vi "Excel_average.vi"(4 "Save?":bool, 6 "1_IL,0_uL":bool, 7 "KG20":dbl[](array[numeric]), 8 "error in (no error)":errorcluster, 9 "Test?":bool, 10 "Report path in":path, 11 "report in":refnum<class "NI_report.lvclass">) -> (0 "error out":errorcluster, 2 "Report path out":path, 3 "report out":refnum<class "NI_report.lvclass">)   [LabVIEW 2015]
doc: "输出电流因数的平均值和与1.125差值"
uses:
  <vilib>/Utility/NIReport.llb/NI_report.lvclass
  <vilib>/addons/_office/NI_ReportGenerationToolkit.lvlib
panel:
  in  "start(-1,-1)":cluster{"row":i32, "column":i32}
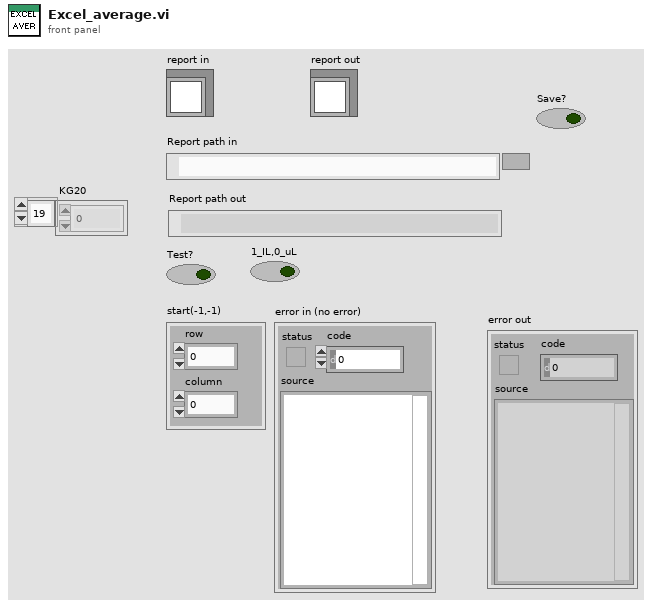
[diagram p1: front panel]
types:
  T1 = enum16{"Standard Report", "HTML", "Word", "Excel"}
  T2 = enum16{"maximized", "minimized", "normal", "no change"}
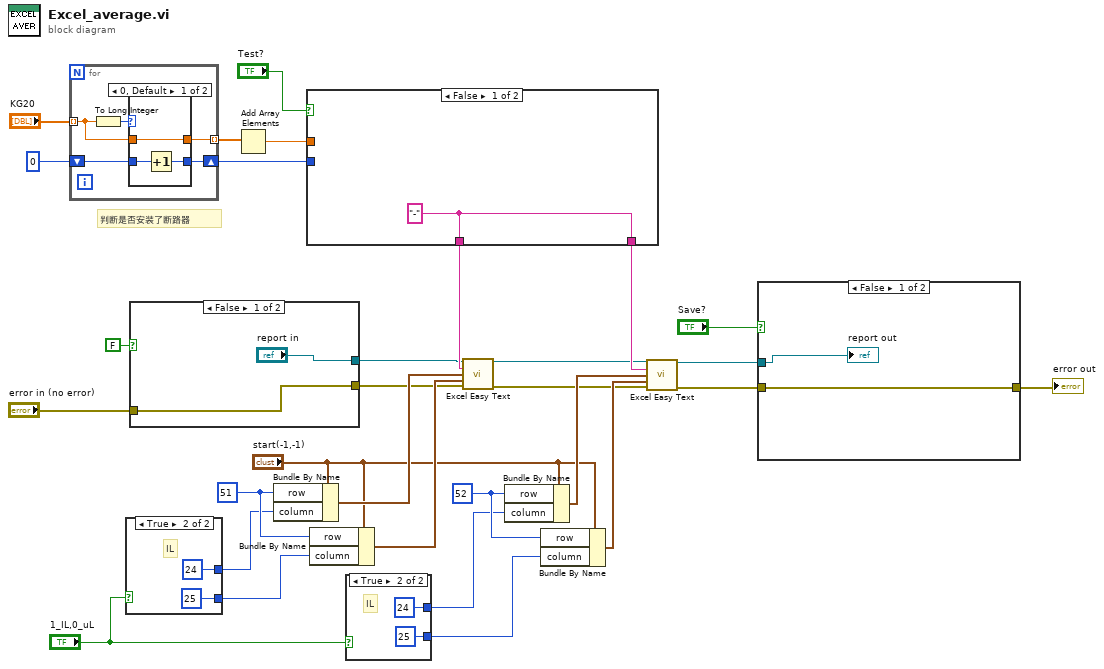
[diagram p0: block diagram]
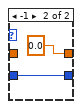
[diagram p2: hidden frame]
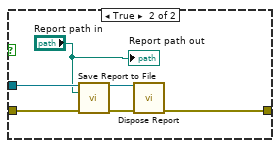
[diagram p3: hidden frame]
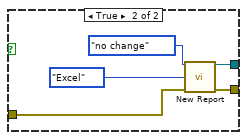
[diagram p4: hidden frame]
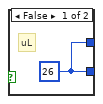
[diagram p5: hidden frame]
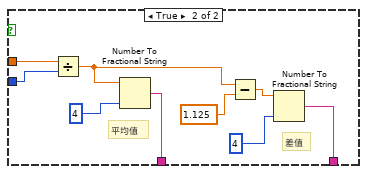
[diagram p6: hidden frame]
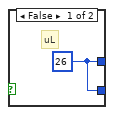
[diagram p7: hidden frame]
diagram:
  w23 = 52 ("row")
  w26 = 51 ("row")
  # "判断是否安装了断路器"
  n1 = for {
    tunnel: "KG20" -> [w33] mode=indexing
    shift-right: [w34] -> w3
    shift-left: 0 -> [w35]
    tunnel: [w32] -> w1 mode=indexing
    n2 = To Long Integer(number=w33) -> (32bit integer=w31:i32)
    n3 = case shown="0, Default" w31 {
      tunnel: w35 -> [w38 w39]
      tunnel: [w36 w39] -> w34
      tunnel: [w37 0.0] -> w32
      tunnel: w33 -> [w37 _]
      frame 0, Default {
        n4 = Increment(x=w38) -> (x+1=w36:i32)
      }
      frame -1 {
      }
    }
  }
  n5 = case shown="True" "1_IL,0_uL" {
    tunnel: [w41 24 ("column")] -> w16
    tunnel: [w41 25 ("column")] -> w15
    frame False {
      w41 = 26 ("column")
      # "uL"
    }
    frame True {
      # "IL"
    }
  }
  n6 = case shown="False" FALSE {
    tunnel: "error in (no error)" -> [w45 w48]
    tunnel: ["report in" w47] -> w25
    tunnel: [w45 w46] -> w24
    frame False {
    }
    frame True {
      n7 = call <vilib>:"New Report.vi"("window state (normal)"=T2."no change", "report type"=T1."Excel", "error in (no error)"=w48) -> ("report out"=w47:refnum<class "NI_report.lvclass">, "error out"=w46:errorcluster)  [unwired: 11 in]
    }
  }
  n8 = Add Array Elements(numeric array=w1) -> (sum=w2:dbl)
  n9 = Bundle By Name(cluster="start(-1,-1)", "row"=w26, "column"=w16) -> (w28:cluster{"row":i32, "column":i32})
  n10 = case shown="False" "Test?" {
    tunnel: [w51 w59] -> w29
    tunnel: w2 -> [_ w57]
    tunnel: [w51 w54] -> w20
    tunnel: w3 -> [_ w52]
    frame False {
      w51 = "-"
    }
    frame True {
      # "差值"
      # "平均值"
      n11 = Divide(x=w57, y=w52) -> (x/y=w53:dbl)
      n12 = Number To Fractional String(number=w53, precision (6)=i16 4) -> (F-format string=w59:string)  [unwired: 2 in]
      n13 = Subtract(x=w53, y=1.125) -> (x-y=w55:dbl)
      n14 = Number To Fractional String(number=w55, precision (6)=i16 4) -> (F-format string=w54:string)  [unwired: 2 in]
    }
  }
  n15 = Bundle By Name(cluster="start(-1,-1)", "row"=w26, "column"=w15) -> (w27:cluster{"row":i32, "column":i32})
  n16 = case shown="True" "1_IL,0_uL" {
    tunnel: [w61 24 ("column")] -> w11
    tunnel: [w61 25 ("column")] -> w10
    frame False {
      w61 = 26 ("column")
      # "uL"
    }
    frame True {
      # "IL"
    }
  }
  n17 = call <vilib>:"Excel Easy Text.vi"("report in"=w25, "text"=w29, "start (-1, -1)"=w28, "end (-1, -1)"=w27, "error in (no error)"=w24) -> ("report out"=w18:refnum<class "NI_report.lvclass">, "error out"=w17:errorcluster)  [unwired: 6 in, 3 out]
  n18 = Bundle By Name(cluster="start(-1,-1)", "row"=w23, "column"=w11) -> (w22:cluster{"row":i32, "column":i32})
  n19 = Bundle By Name(cluster="start(-1,-1)", "row"=w23, "column"=w10) -> (w21:cluster{"row":i32, "column":i32})
  n20 = call <vilib>:"Excel Easy Text.vi"("report in"=w18, "text"=w20, "start (-1, -1)"=w22, "end (-1, -1)"=w21, "error in (no error)"=w17) -> ("report out"=w14:refnum<class "NI_report.lvclass">, "error out"=w13:errorcluster)  [unwired: 6 in, 3 out]
  n21 = case shown="False" "Save?" {
    tunnel: w14 -> [w64 w69]
    tunnel: w13 -> [w65 w68]
    tunnel: [w65 w66] -> w8
    frame False {
      "report out" <- w64
    }
    frame True {
      n22 = call-dynamic "Save Report to File.vi"("report in"=w69, "report file path"="Report path in", "error in (no error)"=w68) -> ("report out"=w71:refnum<class "NI_report.lvclass">, "error out"=w70:errorcluster)  [unwired: 11 in]
      n23 = call-dynamic "Dispose Report.vi"("report in"=w71, "error in (no error)"=w70) -> ("error out"=w66:errorcluster)  [unwired: 13 in]
      "Report path out" <- "Report path in"
    }
  }
  "error out" <- w8
